vi "general_take_PMT_data - Copy.vi"() -> ()   [LabVIEW 2022 SP3]
uses:
  <vilib>/Analysis/NI_AALBase.lvlib
panel:
  out "standard deviation":dbl
  out "mean":dbl
  out "data":u32[](array[numeric])
  out "OLD":bool
  out "DB":u32[](array[numeric])
  out "Overload":i32
  out "Gate Number":i32
  in  "Correction":bool=TRUE
  out "Num Gates Read":i32
  out "Gate Time Read":i32 caption="Gate time Read"
  out "Num Gates Set":i32
  out "Gate Time Set":i32
  out "PowerD":i32 caption="Power\nRead Data"
  out "Handle Number":i32
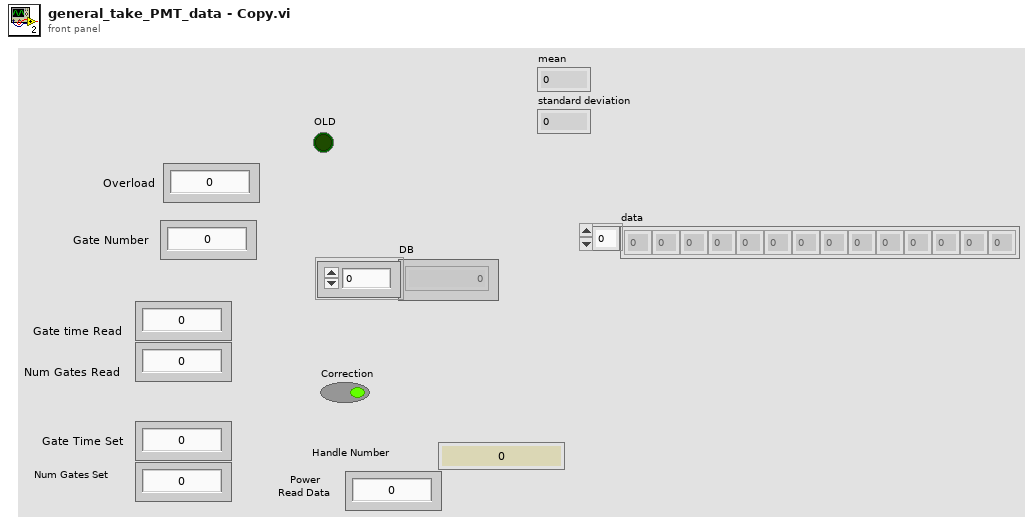
[diagram p1: front panel]
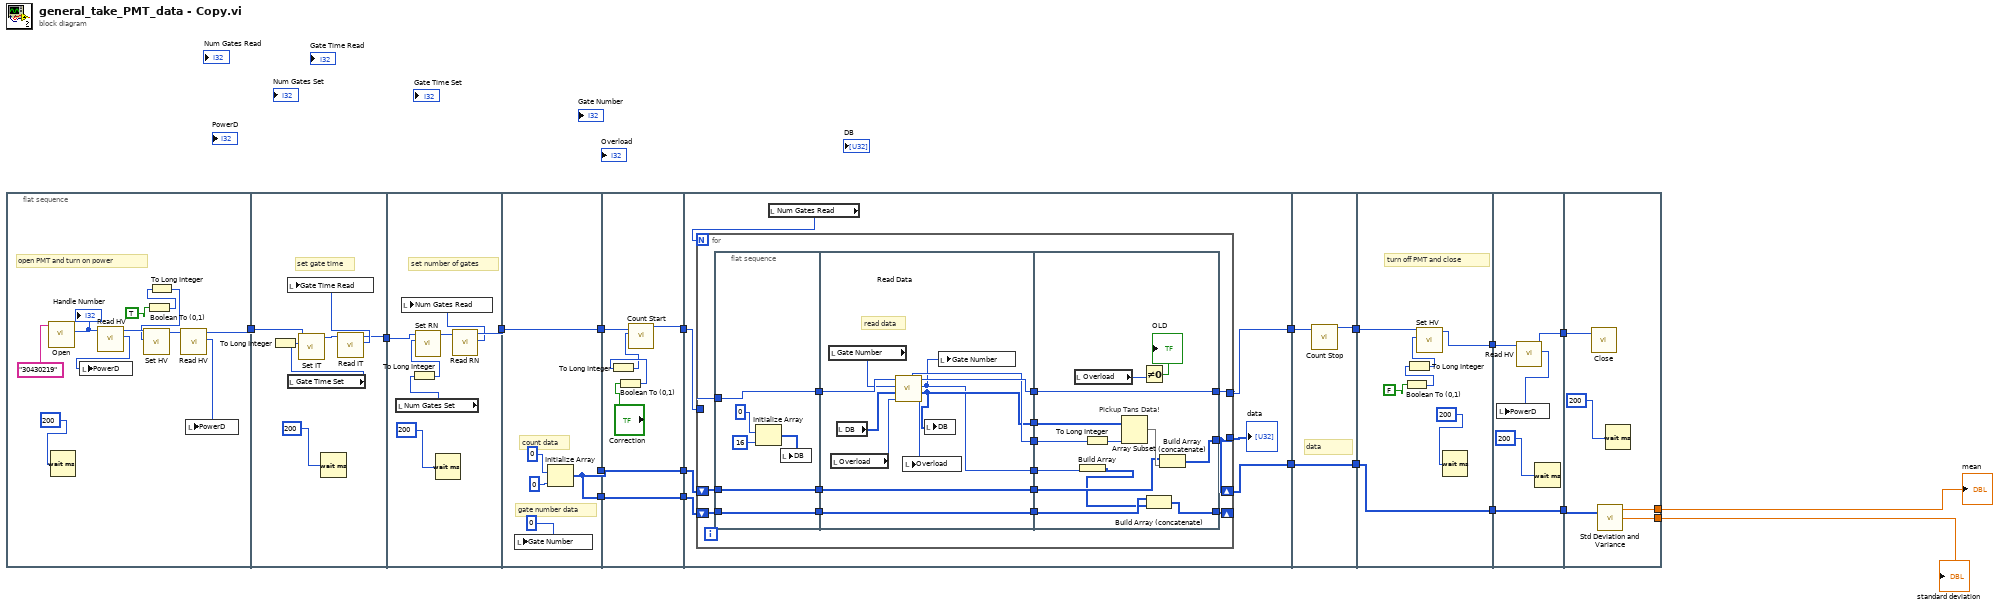
[diagram p0: block diagram]
diagram:
  n1 = flat-sequence {
    tunnel: [w21] -> w19
    tunnel: w19 -> [w37]
    tunnel: [w32] -> w18
    tunnel: [w40] -> w15
    tunnel: w18 -> [w42]
    tunnel: w15 -> [w49]
    tunnel: [w49] -> w3
    tunnel: [w45] -> w2
    tunnel: [w45] -> w1
    tunnel: w3 -> [w56]
    tunnel: [w52] -> w10
    tunnel: w2 -> [w51]
    tunnel: w1 -> [w50]
    tunnel: [w51] -> w9
    tunnel: [w50] -> w8
    tunnel: [w63] -> w17
    tunnel: w10 -> [w62]
    tunnel: w9 -> [w61]
    tunnel: w8 -> [w60]
    tunnel: [w59] -> w13
    tunnel: w17 -> [w111]
    tunnel: [w110] -> w16
    tunnel: [w109] -> w14
    tunnel: w13 -> [w109]
    tunnel: w16 -> [w118]
    tunnel: w14 -> [w112]
    tunnel: [w114] -> w11
    tunnel: [w112] -> w6
    tunnel: [w121] -> w12
    tunnel: w11 -> [w122]
    tunnel: [w119] -> w7
    tunnel: w6 -> [w119]
    tunnel: w12 -> [w128]
    tunnel: w7 -> [w126]
    tunnel: [w125] -> w5
    tunnel: [w124] -> w4
    frame #0 {
      # "open PMT and turn on power"
      n2 = call "Open.vi"("Serial Number"="30430219") -> ("Handle Number"=w29:i32)  [unwired: 9 in, 1 out]
      "Handle Number" <- w29
      n3 = Wait (ms)(milliseconds to wait=u32 200) -> ()  [unwired: 1 out]
      n4 = call "Read HV.vi"("handle"=w29) -> ("HV out"=w27:i32, "handle out"=w28:i32)  [unwired: 8 in, 1 out]
      n5 = local write "PowerD"(w27) -> ()
      n6 = Boolean To (0,1)(Boolean=TRUE) -> (0, 1=w24:i16)
      n7 = To Long Integer(number=w24) -> (32bit integer=w25:i32)
      n8 = call "Set HV.vi"("HV"=w25, "handle"=w28) -> ("handle out"=w23:i32)  [unwired: 8 in, 1 out]
      n9 = call "Read HV.vi"("handle"=w23) -> ("HV out"=w22:i32, "handle out"=w21:i32)  [unwired: 8 in, 1 out]
      n10 = local write "PowerD"(w22) -> ()
    }
    frame #1 {
      # "set gate time"
      n11 = local read "Gate Time Set"() -> (w34:i32)
      n12 = To Long Integer(number=w34) -> (32bit integer=w35:i32)
      n13 = call "Set IT.vi"("IT"=w35, "handle"=w37) -> ("handle out"=w36:i32)  [unwired: 8 in, 1 out]
      n14 = Wait (ms)(milliseconds to wait=u32 200) -> ()  [unwired: 1 out]
      n15 = call "Read IT.vi"("handle"=w36) -> ("IT out"=w33:i32, "handle out"=w32:i32)  [unwired: 8 in, 1 out]
      n16 = local write "Gate Time Read"(w33) -> ()
    }
    frame #2 {
      # "set number of gates"
      n17 = local read "Num Gates Set"() -> (w44:i32)
      n18 = To Long Integer(number=w44) -> (32bit integer=w43:i32)
      n19 = call "Set RN.vi"("RN"=w43, "handle"=w42) -> ("handle out"=w41:i32)  [unwired: 8 in, 1 out]
      n20 = Wait (ms)(milliseconds to wait=u32 200) -> ()  [unwired: 1 out]
      n21 = call "Read RN.vi"("handle"=w41) -> ("RN out"=w39:i32, "handle out"=w40:i32)  [unwired: 8 in, 1 out]
      n22 = local write "Num Gates Read"(w39) -> ()
    }
    frame #3 {
      # "gate number data"
      # "count data"
      n23 = local write "Gate Number"(0) -> ()
      n24 = Initialize Array(u32 0, 0 ("次元サイズ")) -> (w45:u32[])
    }
    frame #4 {
      n25 = Boolean To (0,1)(Boolean="Correction") -> (0, 1=w55:i16)
      n26 = To Long Integer(number=w55) -> (32bit integer=w54:i32)
      n27 = call "Count Start.vi"("Correction"=w54, "handle"=w56) -> ("handle out"=w52:i32)  [unwired: 8 in, 1 out]
    }
    frame #5 {
      n28 = local read "Num Gates Read"() -> (w58:i32)
      n29 = for {
        N: w58 -> [_]
        shift-right: [w64] -> w59
        shift-left: w61 -> [w72]
        shift-right: [w68] -> _
        shift-left: w60 -> [w71]
        tunnel: w62 -> [w73]
        tunnel: [w74] -> w63
        tunnel: [w64] -> w57
        n30 = flat-sequence {
          tunnel: [w84] -> w78
          tunnel: [w83] -> w69
          tunnel: [w82] -> w66
          tunnel: w73 -> [w84]
          tunnel: w72 -> [w83]
          tunnel: w71 -> [w82]
          tunnel: [w95] -> w77
          tunnel: w78 -> [w94]
          tunnel: [w89] -> w76
          tunnel: [w88] -> w75
          tunnel: [w87] -> w70
          tunnel: w69 -> [w87]
          tunnel: [w86] -> w67
          tunnel: w66 -> [w86]
          tunnel: [w85] -> w65
          tunnel: w77 -> [w108]
          tunnel: w76 -> [w103]
          tunnel: w75 -> [w102]
          tunnel: w70 -> [w100]
          tunnel: w67 -> [w99]
          tunnel: w65 -> [w98]
          tunnel: [w108] -> w74
          tunnel: [w101] -> w64
          tunnel: [w96] -> w68
          frame #0 {
            n31 = Initialize Array(u32 0, 16 ("次元サイズ")) -> (w79:u32[])
            n32 = local write "DB"(w79) -> ()
          }
          frame #1 {
            # "read data"
            n33 = local read "Gate Number"() -> (w93:i32)
            n34 = local read "Overload"() -> (w92:i32)
            n35 = local read "DB"() -> (w90:u32[])
            n36 = call "Read Data.vi"("OLD"=w92, "DataBuf"=w90, "GateNum"=w93, "handle"=w94) -> ("OLD out"=w91:i32, "DataBuf out"=w88:u32[], "GateNum out"=w85:i32, "handle out"=w95:i32, "function return"=w89:u32)  [unwired: 3 in]
            n37 = local write "Overload"(w91) -> ()
            n38 = local write "DB"(w88) -> ()
            n39 = local write "Gate Number"(w85) -> ()
          }
          frame #2 {
            # "Pickup Tans Data!"
            n40 = local read "Overload"() -> (w106:i32)
            n41 = Build Array(w98) -> (w97:i32[])
            n42 = To Long Integer(number=w103) -> (32bit integer=w104:i32)
            n43 = Array Subset(array=w102, length=w104) -> (w105:u32[])  [unwired: 1 in]
            n44 = Not Equal To 0?(x=w106) -> (x != 0?=→"OLD":bool)
            n45 = Build Array (concatenate)(w99, w97) -> (w96:u32[])
            n46 = Build Array (concatenate)(w100, w105) -> (w101:u32[])
          }
        }
      }
      "data" <- w57
    }
    frame #6 {
      # "data"
      n47 = call "Count Stop.vi"("handle"=w111) -> ("handle out"=w110:i32)  [unwired: 9 in, 1 out]
    }
    frame #7 {
      # "turn off PMT and close"
      n48 = Boolean To (0,1)(Boolean=FALSE) -> (0, 1=w115:i16)
      n49 = To Long Integer(number=w115) -> (32bit integer=w116:i32)
      n50 = call "Set HV.vi"("HV"=w116, "handle"=w118) -> ("handle out"=w114:i32)  [unwired: 8 in, 1 out]
      n51 = Wait (ms)(milliseconds to wait=u32 200) -> ()  [unwired: 1 out]
    }
    frame #8 {
      n52 = call "Read HV.vi"("handle"=w122) -> ("HV out"=w123:i32, "handle out"=w121:i32)  [unwired: 8 in, 1 out]
      n53 = local write "PowerD"(w123) -> ()
      n54 = Wait (ms)(milliseconds to wait=u32 200) -> ()  [unwired: 1 out]
    }
    frame #9 {
      n55 = call "Close.vi"("Handle"=w128) -> ()  [unwired: 9 in, 2 out]
      n56 = call <vilib>:"Std Deviation and Variance.vi"("X"=w126) -> ("mean"=w125:dbl, "standard deviation"=w124:dbl)  [unwired: 1 in, 1 out]
      n57 = Wait (ms)(milliseconds to wait=u32 200) -> ()  [unwired: 1 out]
    }
  }
  "mean" <- w5
  "standard deviation" <- w4
